vi "Laurel Meter IP Tester.vi"() -> ()   [LabVIEW 2019]
uses:
  Type Definitions/Laurel Serial Commands.ctl
  Type Definitions/Laurel Connection Type.ctl
  Type Definitions/Laurel Display Type.ctl
panel:
  in  "Display Type":T1
  out "Single Item":dbl
  in  "Connection Type":T2
  in  "All Items Byte Count (Flow Rate)":i32=17
  in  "Laurel Serial Commands":T3
  out "return count":i32
  in  "Individual Byte Count":i32=9
  out "Output 5":string="0000.00 0004.71"
  in  "STOP 5":bool
  out "Loop Speed 5":u32
  out "Flow Rate 5":dbl
  out "Gallons 5":dbl
  in  "Error In 6":errorcluster
  out "Error Out 6":errorcluster
  in  "Hot Laurel Only 5":string="10.0.3.167"
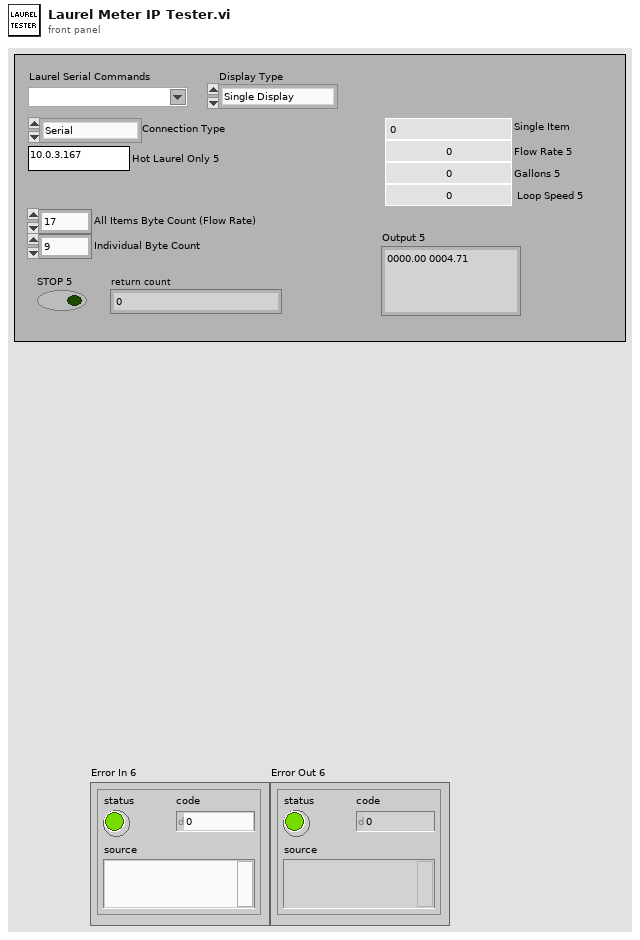
[diagram p1: front panel]
types:
  T1 = typedef "Laurel Display Type.ctl" = enum16{"Single Display", "Dual Display"}
  T2 = typedef "Laurel Connection Type.ctl" = enum16{"Serial", "TCP"}
  T3 = typedef "Laurel Serial Commands.ctl" = string
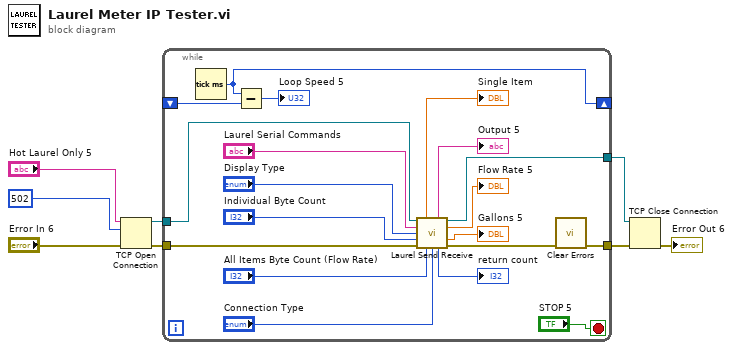
[diagram p0: block diagram]
diagram:
  n1 = TCP Open Connection(address="Hot Laurel Only 5", remote port or service name=u16 502, error in (no error)="Error In 6") -> (connection ID=w5:refnum<k5>, error out=w3:errorcluster)  [unwired: 2 in]
  n2 = while {
    shift-right: [w25] -> _
    shift-left: _ -> [w24]
    tunnel: w3 -> [w21]
    tunnel: [w10] -> w4
    tunnel: w5 -> [w23]
    tunnel: [w22] -> w6
    stop <- "STOP 5" stop-if-true
    n3 = Tick Count (ms)() -> (millisecond timer value=w25:u32)
    n4 = Subtract(x=w25, y=w24) -> (x-y=→"Loop Speed 5":u32)
    n5 = call "Laurel Send Receive.vi"("TCP Network Connection in"=w23, "Laurel Serial Commands"="Laurel Serial Commands", "Display Type"="Display Type", "Individual Byte Count"="Individual Byte Count", "error in (no error)"=w21, "All Items Byte Count (Flow Rate)"="All Items Byte Count (Flow Rate)", "Connection Type"="Connection Type") -> ("Single Item"=→"Single Item":dbl, "Output String"=→"Output 5":string, "TCP Network Connection out"=w22:refnum<k5>, "Flow Rate (Item 1)"=→"Flow Rate 5":dbl, "Gallons (Item 2)"=→"Gallons 5":dbl, "return count"=→"return count":i32, "error out"=w11:errorcluster)  [unwired: 1 in, 1 out]
    n6 = call <vilib>:"Clear Errors.vi"("error in (no error)"=w11) -> ("error out"=w10:errorcluster)  [unwired: 5 in, 1 out]
  }
  n7 = TCP Close Connection(connection ID=w6, error in (no error)=w4) -> (error out=→"Error Out 6":errorcluster)  [unwired: 1 in, 1 out]
